vi "2-Sine Wave Chart (while loop).vi"() -> ()   [LabVIEW 2014]
panel:
  in  "stop":bool
  out "Waveform Chart":dbl(graph)
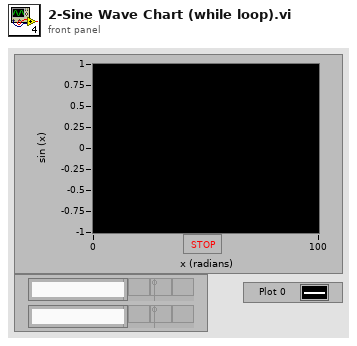
[diagram p1: front panel]
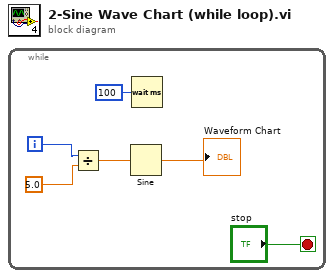
[diagram p0: block diagram]
diagram:
  n1 = while {
    i -> [w2]
    stop <- "stop" stop-if-true
    n2 = Divide(x=w2, y=5.0) -> (x/y=w4:dbl)
    n3 = Sine(x=w4) -> (sin(x)=→"Waveform Chart":dbl)
    n4 = Wait (ms)(milliseconds to wait=u32 100) -> ()  [unwired: 1 out]
  }
